vi "Handle Last Ack Core.vi"(4 "error in":errorcluster, 6 "Last Ack":refnum<class "Last Ack.lvclass">, 7 "SuperActor in":refnum<class "SuperActor.lvclass">) -> (0 "error out":errorcluster, 3 "SuperActor out":refnum<class "SuperActor.lvclass">)   [LabVIEW 2016, in "SuperActor.lvlib" / "SuperActor.lvclass"]
doc: "(<B>Filename</B>: Actor Framework.lvlib:Actor.lvclass:Handle Last Ack Core.vi)\n\nDefines how the caller actor responds to the Last Ack message from a nested actor. The Last Ack message is the final message a nested actor sends to its caller before it shuts down. The message contains information about the final state of the nested actor.\n\nBy default, this method does nothing except return any error the nested actor sent. A descendant class may override this method to define behavior."
uses:
  SuperActor.lvclass
  <vilib>/ActorFramework/LastAck/Last Ack.lvclass
  C:/Program Files (x86)/National Instruments/LabVIEW 2016/vi.lib/ActorFramework/Actor/Actor.lvclass
  <vilib>/ActorFramework/LastAck/Last Ack.lvclass/Last Ack.ctl
  SuperActor.lvclass/SuperActor.ctl
  <vilib>/ActorFramework/Actor/Actor.lvclass/Actor.ctl
  <vilib>/ActorFramework/Message Enqueuer/Message Enqueuer.lvclass/Message Enqueuer.ctl
  Read ID.vi
  <vilib>/ActorFramework/Message Enqueuer/Init from Existing Queue.vi
  <vilib>/ActorFramework/Message Enqueuer/Enqueue.vi
  <vilib>/ActorFramework/Stop Msg/Stop Msg.lvclass
  C:/Program Files (x86)/National Instruments/LabVIEW 2016/vi.lib/ActorFramework/Message/Message.lvclass
  <vilib>/ActorFramework/Message Priority Queue/Priority Enqueue.vi
  <vilib>/ActorFramework/Message Enqueuer/Message Enqueuer.lvclass
  Session APIs/Session Log/System Log.lvclass
  <vilib>/ActorFramework/Actor/Actor.lvclass
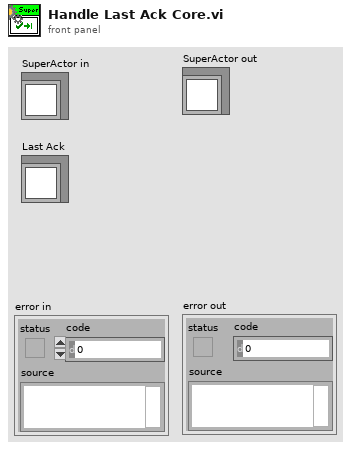
[diagram p1: front panel]
types:
  T1 = typedef "Session - Root.lvclass/Session Handle.ctl" = refnum<data-value>
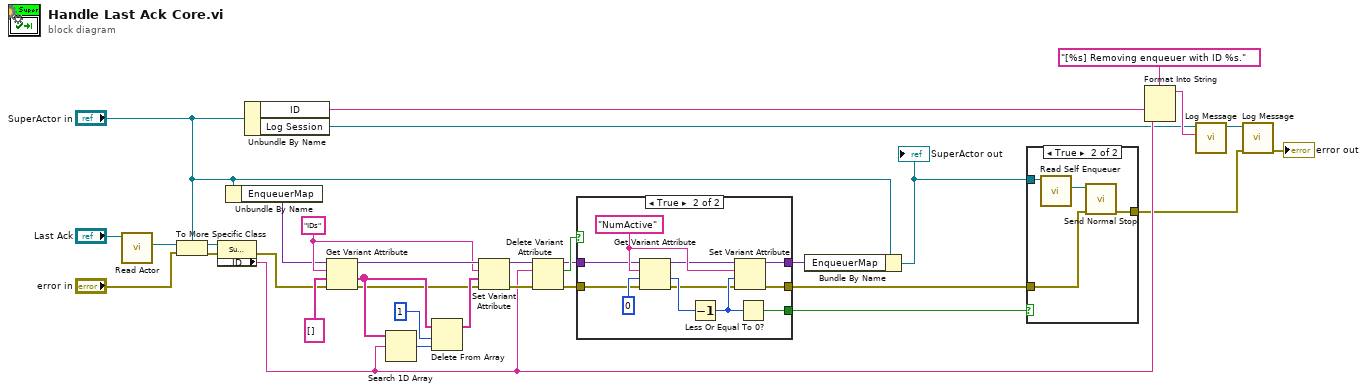
[diagram p0: block diagram]
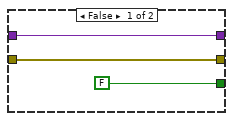
[diagram p3: hidden frame]
diagram:
  w25 = "IDs" ("name")
  n1 = call <vilib>:"Read Actor.vi"("Last Ack"="Last Ack") -> ("Actor"=w33:refnum<class "Actor.lvclass">)  [unwired: 10 in]
  n2 = To More Specific Class(target class="SuperActor in", reference=w33, error in="error in") -> (specific class reference=w17:refnum<class "SuperActor.lvclass">, error out=w15:errorcluster)
  n3 = property class="SuperActor"(reference=w17, error in=w15) -> (error out=w16:errorcluster, "Accessors:ID"=w11:string)  [unwired: 1 out]
  n4 = Unbundle By Name("SuperActor in") -> ("EnqueuerMap"=w1:variant)
  n5 = Unbundle By Name("SuperActor in") -> ("ID"=w5:string, "Log Session"=w4:T1)
  n6 = Get Variant Attribute(Variant=w1, name=w25, default value (empty Variant)=string[] [], error in=w16) -> (duplicate Variant=w27:variant, value=w28:string[], error out=w23:errorcluster)  [unwired: 1 out]
  n7 = Search 1D Array(1D array=w28, element=w11) -> (index of element=w29:i32)  [unwired: 1 in]
  n8 = Delete From Array(array=w28, length=1, index=w29) -> (array with subset deleted=w26:string[])  [unwired: 1 out]
  n9 = Set Variant Attribute(Variant=w27, name=w25, value=w26, error in=w23) -> (Variant out=w22:variant, error out=w21:errorcluster)  [unwired: 1 out]
  n10 = Delete Variant Attribute(4:w21, 6:w11, 7:w22) -> (0:w19:errorcluster, 2:w20:bool, 3:w18:variant)
  n11 = case shown="True" w20 {
    tunnel: [FALSE w41] -> w14
    tunnel: w18 -> [w34 w40]
    tunnel: w19 -> [w36 w39]
    tunnel: [w36 w38] -> w12
    tunnel: [w34 w37] -> w6
    frame False {
    }
    frame True {
      w45 = "NumActive" ("name")
      n12 = Get Variant Attribute(Variant=w40, name=w45, default value (empty Variant)=i16 0, error in=w39) -> (duplicate Variant=w42:variant, value=w47:i16, error out=w43:errorcluster)  [unwired: 1 out]
      n13 = Decrement(x=w47) -> (x-1=w44:i16)
      n14 = Set Variant Attribute(Variant=w42, name=w45, value=w44, error in=w43) -> (Variant out=w37:variant, error out=w38:errorcluster)  [unwired: 1 out]
      n15 = Less Or Equal To 0?(x=w44) -> (x <= 0?=w41:bool)
    }
  }
  n16 = Bundle By Name(cluster="SuperActor in", "EnqueuerMap"=w6) -> (w3:refnum<class "SuperActor.lvclass">)
  "SuperActor out" <- w3
  n17 = case shown="True" w14 {
    tunnel: w3 -> [_ w50]
    tunnel: w12 -> [w48 w52]
    tunnel: [w48 w51] -> w8
    frame False {
    }
    frame True {
      n18 = call <vilib>:"Read Self Enqueuer.vi"("Actor"=w50) -> ("Self Enqueuer"=w49:refnum<class "Message Enqueuer.lvclass">)  [unwired: 10 in]
      n19 = call <vilib>:"Send Normal Stop.vi"("error in (no error)"=w52, "Message Enqueuer"=w49) -> ("error out"=w51:errorcluster)  [unwired: 9 in]
    }
  }
  n20 = Format Into String(format string="[%s] Removing enqueuer with ID %s.", w5, w11) -> (resulting string=w10:string)  [unwired: 2 in, 1 out]
  n21 = call "Log Message.vi"("MSG In"=w10, "session in"=w4) -> ("session out"=w9:T1)  [unwired: 8 in, 1 out]
  n22 = call "Log Message.vi"("error in"=w8, "session in"=w9) -> ("error out"=→"error out":errorcluster)  [unwired: 8 in, 1 out]
